vi "Creators Creator Queue Alias.vi"(11 "Base Event in":refnum<class "Base Event.lvclass">) -> (2 "Creator Queue Alias":string, 3 "Base Event out":refnum<class "Base Event.lvclass">)   [LabVIEW 2021, in "jettl.lvlib" / "Base Event.lvlib" / "Base Event.lvclass"]
uses:
  Base Event.lvclass
  C:/git/jettl/jettl/jettl/jettl/jettl.lvclass
  Base Event.lvclass/Base Event.ctl
  Addresses/Addresses.lvlib
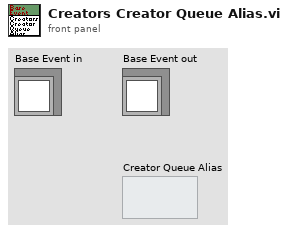
[diagram p1: front panel]
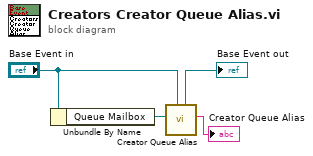
[diagram p0: block diagram]
diagram:
  n1 = Unbundle By Name("Base Event in") -> ("Queue Mailbox"=w4:refnum<data-value>)
  n2 = call "Creator Queue Alias.vi"("jettl in"="Base Event in", "Queue Mailbox"=w4) -> ("Creator Queue Alias"=→"Creator Queue Alias":string, "jettl out"=→"Base Event out":refnum<class "Base Event.lvclass">)  [unwired: 8 in]
